vi "VI to XML.vi"(7 "VI Path":string) -> (0 "Error Out":errorcluster, 2 "Conversion Messages":string[](array[string]), 3 "XML (UTF-8 encoded)":string="<VI _name=\"volume1.vi\">\n  <Control _name=\"radius\" conIdx=\"11\" value=\"T10:0\"/>\n  <Constant outputs=\"four\" value=\"T10:4\"/>\n  <Constant outputs=\"three\" value=\"T10:3\"/>\n  <FixedConst _name=\"PI\" outputs=\"pi\"/>\n  <Multiply inputs=\"radius;radius\" outputs=\"x*y\"/>\n  <Multiply inputs=\"x*y;radius\" outputs=\"x*y2\"/>\n  <Multiply inputs=\"x*y2;four\" outputs=\"x*y3\"/>\n  <Divide inputs=\"x*y3;three\" outputs=\"x/y\"/>\n  <Multiply inputs=\"x/y;pi\" outputs=\"volume\"/>\n  <Indicator _name=\"volume\" conIdx=\"3\" value=\"T10:0\"/>\n</VI>")   [LabVIEW 2026]
uses:
  LV AI Core/LV AI Core.lvlib
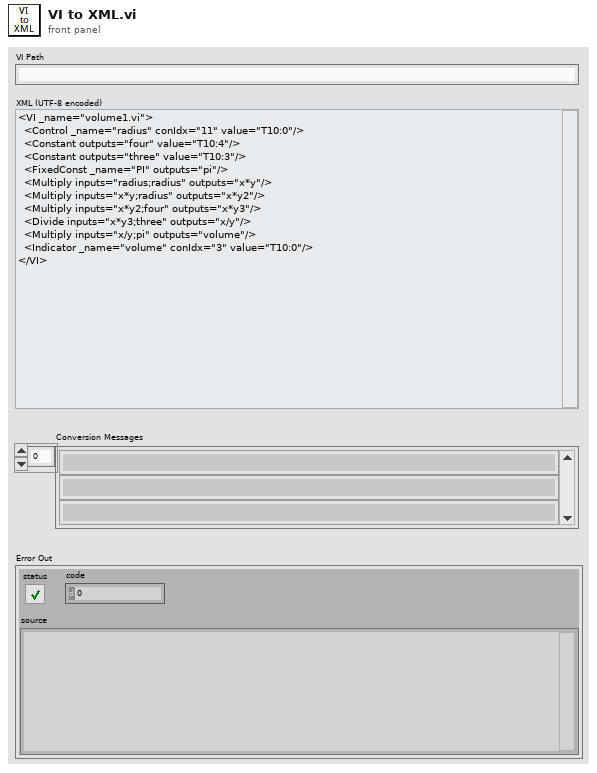
[diagram p1: front panel]
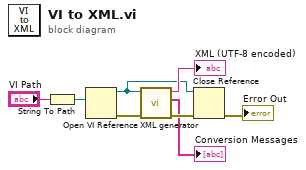
[diagram p0: block diagram]
diagram:
  n1 = String To Path(string="VI Path") -> (path=w2:path)
  n2 = Open VI Reference(vi path=w2) -> (vi reference=w3:refnum<vi>, error out=w8:errorcluster)  [unwired: 5 in]
  n3 = call "XML generator.vi"("error in (no error)"=w8, "vi"=w3) -> ("error out"=w5:errorcluster, "conversion messages"=→"Conversion Messages":string[], "XML (UTF-8 encoded)"=→"XML (UTF-8 encoded)":string)  [unwired: 6 in, 1 out]
  n4 = Close Reference(reference=w3, error in (no error)=w5) -> (error out=→"Error Out":errorcluster)
